vi "RT Main.vi"() -> ()   [LabVIEW 2014]
uses:
  <vilib>/addons/_NISVFA/_Shared subVIs/Controls/svc_Window.ctl
  <vilib>/addons/_NISVFA/_Shared subVIs/Controls/svc_Channel Info.ctl
  <vilib>/addons/_NISVFA/_Shared subVIs/Controls/svc_Engineering Units Text Ring.ctl
  <vilib>/addons/_NISVFA/_Shared subVIs/Controls/svc_Weighting Filter Text Ring.ctl
  <vilib>/NI/cRIO Wfm/ChannelConfig.ctl
  <vilib>/addons/Sound and Vibration/svt_Calibration/SVL Scale Voltage to EU (N Ch - 1 Info).vi
  <vilib>/addons/Sound and Vibration/svt_Calibration/SVL Scale Voltage to EU (1 Ch).vi
  <vilib>/addons/_NISVFA/_Shared subVIs/Common/svc_Set SV Channel Info.vi
  <vilib>/addons/_NISVFA/_Shared subVIs/Common/svc_Set SV Channel Info (variant).vi
  <vilib>/addons/_NISVFA/_Shared subVIs/Common/SVL Set dB Reference (variant).vi
  <vilib>/FPGAPlugInAG/sbRIO-9651/niLvFpga_Open_sbRIO-9651.vi
  <vilib>/rvi/interface/common/dynamic/niFpgaDynamicAddResources.vi
  <vilib>/FPGAPlugInAG/Dynamic/niLvFpga_Reset_Dynamic.vi
  <vilib>/FPGAPlugInAG/Dynamic/niLvFpga_Run_Dynamic.vi
  <vilib>/NI/cRIO Wfm/AcqRead(Wfm).vi
  <vilib>/addons/_NISVFA/_Shared subVIs/Common/svc_Engineering Units to Unit Label.vi
  <vilib>/addons/_NISVFA/_Shared subVIs/Common/svc_Compute Scale Factor to Convert V to EU.vi
  <vilib>/addons/_NISVFA/_Shared subVIs/Common/svc_Set dB ref if Pascal.vi
  <vilib>/addons/_NISVFA/_Shared subVIs/Common/svc_Caller VI Returned in Error Source.vi
  <vilib>/addons/_NISVFA/_Baseband FFT/SVFA Power Spectrum (N Ch).vi
  <vilib>/addons/_NISVFA/_Zoom FFT/SVFA Zoom Power Spectrum (N Ch).vi
  <vilib>/addons/_NISVFA/_Subset FFT/SVFA Power Spectrum Subset (N Ch).vi
  <vilib>/addons/_NISVFA/_Baseband FFT/SVFA FFT Spectrum (Mag-Phase) (N Ch).vi
  <vilib>/addons/_NISVFA/_Zoom FFT/SVFA Zoom FFT Spectrum (Mag-Phase) (N Ch).vi
  <vilib>/addons/_NISVFA/_Subset FFT/SVFA FFT Spectrum Subset (Mag-Phase) (N Ch).vi
  <vilib>/addons/_NISVFA/_Baseband FFT/SVFA Power Spectral Density (N Ch).vi
  <vilib>/addons/_NISVFA/_Zoom FFT/SVFA Zoom Power Spectral Density (N Ch).vi
  <vilib>/addons/_NISVFA/_Subset FFT/SVFA Power Spectral Density Subset (N Ch).vi
  <vilib>/FPGAPlugInAG/Dynamic/niLvFpga_Close_Dynamic.vi
  <vilib>/rvi/interface/nirviOpenFPGA/nirviOpenFPGA.xnode
  FPGA Bitfiles/SOMHands-ON_FPGATarget_FPGAMainSPIAPIwi_O70J1gyptM8.lvbitx
  FPGA Main_SPI API with Waveform Library.vi
  <vilib>/rvi/interface/nirviMethod/nirviMethod.xnode
  <vilib>/rvi/interface/nirviCloseFPGA/nirviCloseFPGA.xnode
  <vilib>/NI/cRIO Wfm/cRIO Wfm.lvlib
  <vilib>/addons/Sound and Vibration/svt_Calibration/SoundVib_Calibration.lvlib
panel:
  in  "channel info":T1={"sensor sensitivity [mV/EU]"=1000.0, "engineering units"=1, "dB reference [EU]"=1.0, "custom label"="EU", "weighting filter"=0, "pregain [dB]"=0.0} {"pregain [dB]" format="%.2f"; "weighting filter" items=["Linear", "A-weighting", "B-weighting", "C-weighting", "ITU-R 468-4", "Dolby", "CCITT", "C-message", "Wb", "Wc", "Wd", "We", "Wf", "Wh", "Wj", "Wk", "Wm", "AES17 20 kHz lowpass", "AES17 40 kHz lowpass", "AES17 20 kHz highpass", "AES17 40 kHz highpass"]; "dB reference [EU]" format="%^.1e"; "engineering units" items=["custom..."=0, "V"=1, "A"=21, "Pa"=2, "N"=20, "g"=3, "m/s^2"=4, "m/s"=5, "m"=6, "mm/s"=12, "mm"=13, "micron/s"=14, "micron"=15, "in/s^2"=7, "in/s"=8, "in"=9, "mil/s"=10, "mil"=11, "rad/s^2"=16, "rad/s"=17, "rad"=18, "deg/s^2"=26, "deg/s"=27, "deg"=28, "RPM"=22, "cycle/s^2"=23, "Hz"=24, "cycle"=25, "strain"=19]; "sensor sensitivity [mV/EU]" format="%.2f"}
  in  "scan rate [S/s]":u32=25000
  in  "quit":bool
  in  "window":T4=1 items=["None"=0, "Hanning"=1, "Hamming"=2, "Blackman-Harris"=3, "Exact Blackman"=4, "Blackman"=5, "Flat Top"=6, "4 Term B-Harris "=7, "7 Term B-Harris"=8, "Low Sidelobe"=9, "Force"=64, "Exponential"=65, "Blackman Nuttall"=11, "Triangle"=30, "Bartlett-Hanning"=31, "Bohman"=32, "Parzen"=33, "Welch"=34, "Kaiser"=60, "Dolph-Chebyshev"=61, "Gaussian"=62]
  in  "Graph Tab Control":T5(tab)
  out "Power spectrum":cluster{"f0":dbl, "df":dbl, "magnitude":dbl[]}[](graph)
  out "Phase":cluster{"f0":dbl, "df":dbl, "phase":dbl[]}[](graph)
  out "Magnitude":cluster{"f0":dbl, "df":dbl, "magnitude":dbl[]}[](graph)
  out "PSD":cluster{"f0":dbl, "df":dbl, "magnitude":dbl[]}[](graph)
  in  "dB On":bool=TRUE
  in  "FFT Type":enum32{"Baseband", "Zoom", "Subset"}(tab)
  out "frequency resolution [Hz]":dbl=50.0 format="%.2f"
  out "time record [ms]":dbl=20.0 format="%.2f"
  in  "zoom settings":T6={"frequency range"={"start frequency"=500.0, "stop frequency"=2000.0}, "window"=enum."Hanning", "number of lines"=400, "% overlap"=0.0} {"% overlap" min=0.0 max=99.0 step=10.0 format="%.2f"; "number of lines" min=1 step=1; "frequency range"."stop frequency" min=0.0 format="%.2f"; "frequency range"."start frequency" min=0.0 format="%.2f"}
  out "zoom FFT":dbl=2.500000055879356 format="%.2f"
  out "baseband FFT":dbl=50.0 format="%.2f"
  out "frequency resolution [Hz] Subset":dbl format="%.2f"
  out "time record [ms] Subset":dbl format="%.2f"
  in  "frequency range 2":T7={"start frequency"=200.0, "stop frequency"=2000.0} {"stop frequency" min=0.0 format="%.2f"; "start frequency" min=0.0 format="%.2f"}
  in  "number of samples":i32=2000 min=128
  out "averages completed":dbl
  out "done":bool
  in  "averaging mode":T8(ring)=enum."RMS averaging"
  in  "number of averages":u32=10
  in  "linear mode":enum16{"One shot", "Auto restart"}(ring)=enum."Auto restart"
  in  "weighting mode":enum16{"Linear", "Exponential"}(ring)=enum."Exponential"
  in  "restart 2":bool
  in  "Samples per Channel":i32=1000
  # "Channel Settings"
  # "Averaging Settings"
  # "Analysis Settings"
  # "VI Controls"
  # "Increase number of samples to improve frequency resolution (for a given sampling frequency)"
  # "frequency resolution [Hz]"
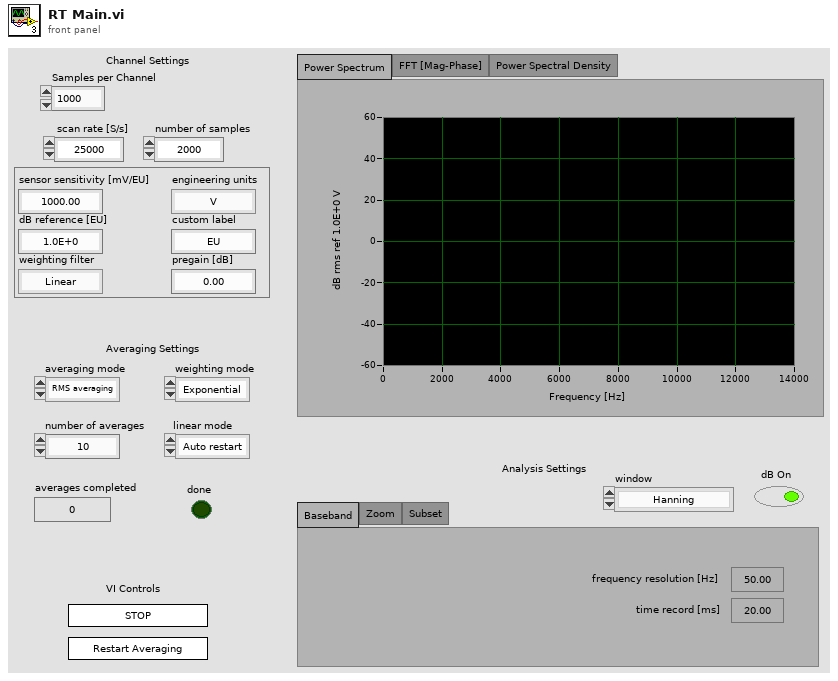
[diagram p1: front panel]
types:
  T1 = typedef "svc_Channel Info.ctl" = cluster{"sensor sensitivity [mV/EU]":dbl, "engineering units":T2, "dB reference [EU]":dbl, "custom label":string, "weighting filter":T3, "pregain [dB]":dbl}
  T2 = typedef "svc_Engineering Units Text Ring.ctl" = u16
  T3 = typedef "svc_Weighting Filter Text Ring.ctl" = u16
  T4 = typedef "svc_Window.ctl" = u32
  T5 = enum32{"Power Spectrum", "FFT [Mag-Phase]", "Power Spectral Density"}
  T6 = cluster{"frequency range":cluster{"start frequency":dbl, "stop frequency":dbl}, "window":enum16{"None ", "Hanning", "Hamming", "Blackman-Harris", "Exact Blackman", "Blackman", "Flat Top", "4 Term B-Harris ", "7 Term B-Harris", "Low Sidelobe"}, "number of lines":i32, "% overlap":dbl}
  T7 = cluster{"start frequency":dbl, "stop frequency":dbl}
  T8 = enum16{"No averaging", "Vector averaging", "RMS averaging", "Peak hold"}
  T9 = typedef "cRIO Wfm.lvlib/ChannelConfig.ctl" = cluster{"Channel Name":string, "Sensitivity mV_EU":dbl, "EU":string, "dB Ref EU":dbl}[]
  T10 = typedef "cRIO Wfm.lvlib/SamplingInfo.ctl" = cluster{"Number of Channels":i32, "Actual Samp Rate":dbl, "Chan Name Array":string[], "EU Chan Array":string[], "dB Ref Chan Array":dbl[]}
  T11 = cluster{"averaging mode":enum16{"No averaging", "Vector averaging", "RMS averaging", "Peak hold"}, "weighting mode":enum16{"Linear", "Exponential"}, "number of averages":u32, "linear mode":enum16{"One shot", "Auto restart"}}
  T12 = cluster{"dB On (T)":bool, "unwrap phase (F)":bool, "convert to degree (T)":bool}
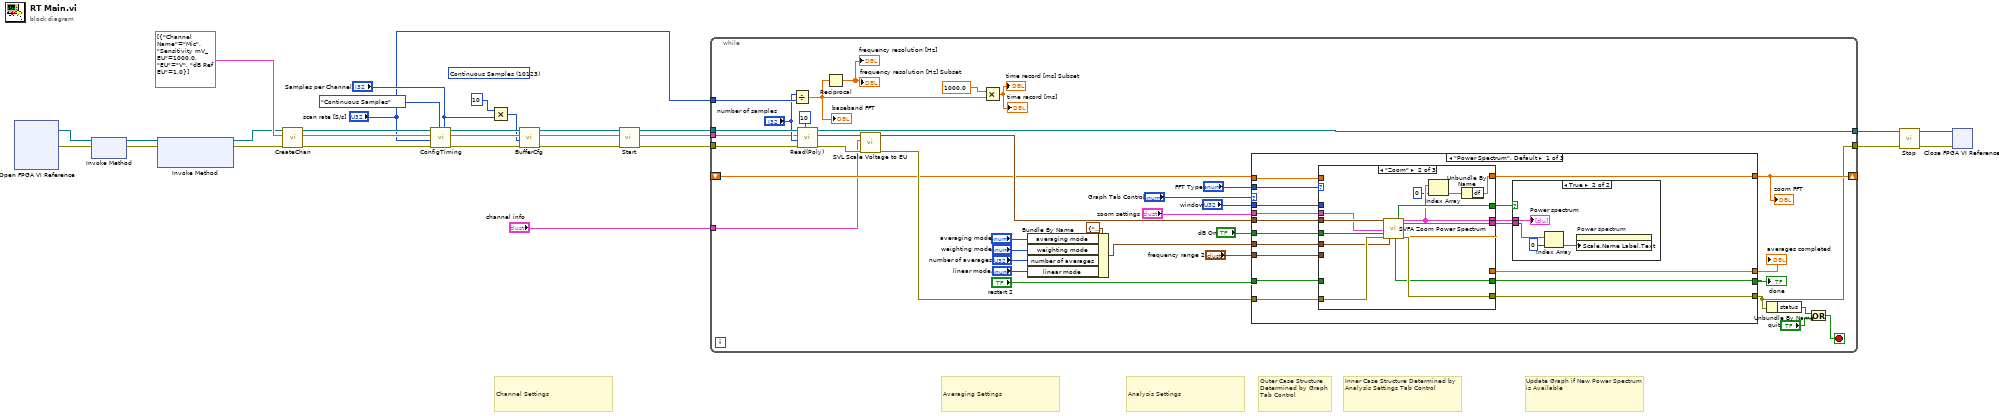
[diagram p0: block diagram]
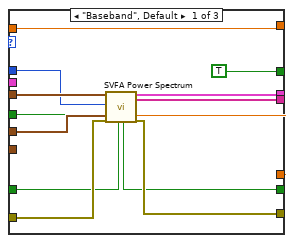
[diagram p3: hidden frame]
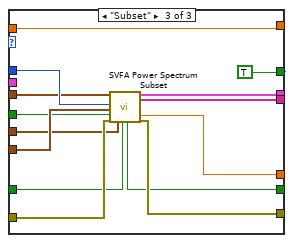
[diagram p4: hidden frame]
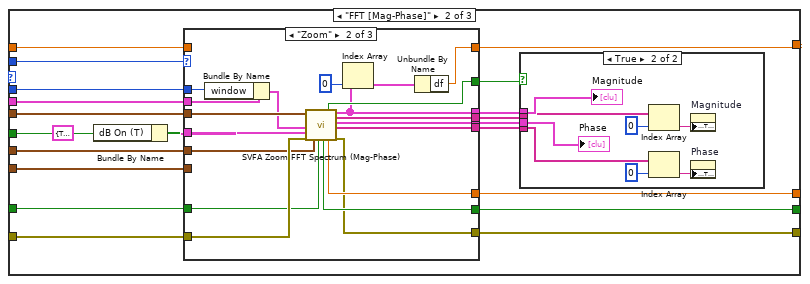
[diagram p5: hidden frame]
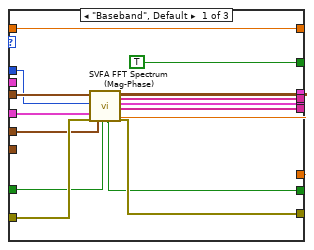
[diagram p7: hidden frame]
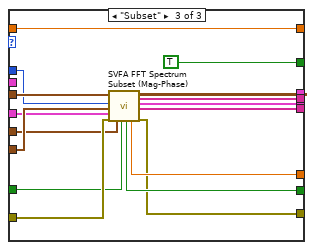
[diagram p8: hidden frame]
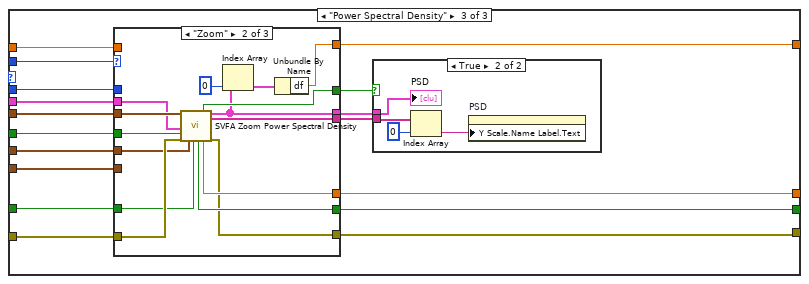
[diagram p9: hidden frame]
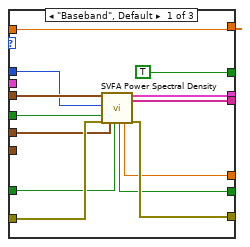
[diagram p11: hidden frame]
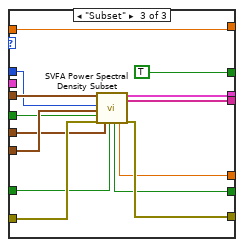
[diagram p12: hidden frame]
diagram:
  (unwired) 10123 items=["Finite Samples"=10178, "Continuous Samples"=10123] ("sample mode")
  # "Channel Settings"
  # "Update Graph if New Power Spectrum is Available"
  # "Inner Case Structure Determined by Analysis Settings Tab Control"
  # "Analysis Settings"
  # "Outer Case Structure Determined by Graph Tab Control"
  # "Averaging Settings"
  n1 = xnode "Open FPGA VI Reference"() -> ("FPGA VI Reference Out"=w15:refnum<k20>, "error out"=w16:errorcluster)  [unwired: 2 in]
  n2 = xnode "Invoke Method"("FPGA VI Reference In"=w15, "error in"=w16) -> ("FPGA VI Reference Out"=w14:refnum<k20>, "error out"=w11:errorcluster)
  n3 = xnode "Invoke Method"("FPGA VI Reference In"=w14, "error in"=w11) -> ("FPGA VI Reference Out"=w13:refnum<k20>, "error out"=w12:errorcluster)  [unwired: 1 in]
  n4 = call <vilib>:"CreateChan.vi"("error in"=w12, "Channel Info"=T9 [{"Channel Name"="Mic", "Sensitivity mV_EU"=1000.0, "EU"="V", "dB Ref EU"=1.0}], "Dynamic FPGA Ref"=w13) -> ("error out"=w19:errorcluster, "Sampling Info"=w23:T10, "Dynamic FPGA Ref Out"=w29:refnum<k20>)  [unwired: 6 in]
  n5 = call <vilib>:"ConfigTiming.vi"("Samples per Channel"="Samples per Channel", "Sample Mode"=enum16{"Finite Samples", "Continuous Samples"}."Continuous Samples", "error in"=w19, "Sample Rate"="scan rate [S/s]", "Sampling Info In"=w23, "Dynamic FPGA Ref"=w29) -> ("error out"=w18:errorcluster, "Sampling Info Out"=w24:T10, "Dynamic FPGA Ref Out"=w28:refnum<k20>)  [unwired: 2 in, 1 out]
  n6 = Multiply(x=10, y="Samples per Channel") -> (x*y=w20:i32)
  n7 = call <vilib>:"BufferCfg.vi"("error in"=w18, "Buffer Size [Samps per Chan]"=w20, "Sampling Info In"=w24, "Dynamic FPGA Ref"=w28) -> ("error out"=w17:errorcluster, "Sampling Info Out"=w22:T10, "Dynamic FPGA Ref Out"=w27:refnum<k20>)  [unwired: 4 in, 1 out]
  n8 = call <vilib>:"Start.vi"("error in"=w17, "Sampling Info In"=w22, "Dynamic FPGA Ref"=w27) -> ("error out"=w2:errorcluster, "Sampling Info Out"=w1:T10, "Dynamic FPGA Ref Out"=w3:refnum<k20>)  [unwired: 6 in]
  n9 = while {
    tunnel: [w32] -> w5
    shift-right: [w53] -> _
    shift-left: _ -> [w56]
    tunnel: [w48] -> w6
    tunnel: w3 -> [w47]
    tunnel: "scan rate [S/s]" -> [w46]
    tunnel: w2 -> [w43]
    tunnel: "channel info" -> [w34]
    tunnel: w1 -> [w30]
    stop <- w65 stop-if-true
    n10 = Divide(x="number of samples", y=w46) -> (x/y=w54:dbl)
    "baseband FFT" <- w54
    n11 = call-poly <vilib>:"Read(Poly).vi"("Poll Time (ms)"=u32 10, "error in"=w43, "Samps Read per Chan"="number of samples", "Sampling Info"=w30, "Dynamic FPGA Ref"=w47) -> ("error out"=w44:errorcluster, "Wfm Data"=w49:waveform(sgl)[], "Dynamic FPGA Ref Out"=w48:refnum<k20>)  [unwired: 3 in, 1 out]
    n12 = Reciprocal(x=w54) -> (1/x=→"frequency resolution [Hz]" →"frequency resolution [Hz] Subset":dbl)
    n13 = call-poly <vilib>:"SVL Scale Voltage to EU.vi"("error in (no error)"=w44, "channel info"=w34, "signals [V]"=w49) -> ("error out"=w64:errorcluster, "scaled signals [EU]"=w63:waveform(dbl)[])  [unwired: 6 in, 1 out]
    n14 = Multiply(x=1000.0 ("y"), y=w54) -> (x*y=→"time record [ms]" →"time record [ms] Subset":dbl)
    n15 = Bundle By Name(cluster=T11 {"averaging mode"=enum."RMS averaging", "weighting mode"=enum."Exponential", "number of averages"=10, "linear mode"=enum."Auto restart"} ("averaging parameters"), "averaging mode"="averaging mode", "weighting mode"="weighting mode", "number of averages"="number of averages", "linear mode"="linear mode") -> (w37:T11)
    n16 = case shown="\"Power Spectrum\", Default" "Graph Tab Control" {
      tunnel: w64 -> [w82 w149 w223]
      tunnel: w63 -> [w83 w148 w224]
      tunnel: [w81 w147 w222] -> w32
      tunnel: "window" -> [w80 w131 w221]
      tunnel: w37 -> [w79 w146 w220]
      tunnel: "restart 2" -> [w78 w145 w208]
      tunnel: [w76 w144 w219] -> w35
      tunnel: [w75 w143 w218] -> w36
      tunnel: "dB On" -> [w74 w141 w212]
      tunnel: "FFT Type" -> [w72 w136 w214]
      tunnel: [w71 w133 w211] -> w53
      tunnel: w56 -> [w69 w132 w210]
      tunnel: "zoom settings" -> [w68 w135 w213]
      tunnel: "frequency range 2" -> [w67 w130 w209]
      frame "Power Spectrum", Default {
        n17 = case shown="\"Zoom\"" w72 {
          tunnel: w83 -> [w100 w114 w126]
          tunnel: w82 -> [w99 w113 w125]
          tunnel: [w98 w112 w123] -> w81
          tunnel: w80 -> [w97 _ w127]
          tunnel: w79 -> [w96 w101 w115]
          tunnel: w78 -> [w95 _ w117]
          tunnel: [w94 w103 w124] -> w77
          tunnel: [w93 w107 w118] -> w76
          tunnel: [w92 w106 w119] -> w75
          tunnel: w74 -> [w91 w105 w116]
          tunnel: [w90 w109 w122] -> w73
          tunnel: [w88 w111 w120] -> w71
          tunnel: [TRUE ("new spectrum available") w110 TRUE ("new spectrum available")] -> w70
          tunnel: w69 -> [w88 _ w120]
          tunnel: w68 -> [_ w108 _]
          tunnel: w67 -> [_ _ w128]
          frame "Baseband", Default {
            n18 = call-poly <vilib>:"SVFA Power Spectrum.vi"("scaled signals [EU]"=w100, "window"=w97, "dB On (T)"=w91, "error in (no error)"=w99, "averaging parameters"=w96, "restart averaging (F)"=w95) -> ("averaging done"=w93:bool, "averages completed"=w92:dbl, "power spectra [dB EU]"=w94:cluster{"f0":dbl, "df":dbl, "magnitude":dbl[]}[], "unit labels"=w90:string[], "error out"=w98:errorcluster)  [unwired: 8 in, 1 out]
          }
          frame "Zoom" {
            n19 = call-poly <vilib>:"SVFA Zoom Power Spectrum.vi"("scaled signals [EU]"=w114, "zoom settings"=w108, "dB On (T)"=w105, "error in (no error)"=w113, "averaging parameters"=w101) -> ("averaging done"=w107:bool, "new spectrum available"=w110:bool, "averages completed"=w106:dbl, "power spectra [dB EU]"=w103:cluster{"f0":dbl, "df":dbl, "magnitude":dbl[]}[], "unit labels"=w109:string[], "error out"=w112:errorcluster)  [unwired: 8 in, 1 out]
            n20 = Index Array(array=w103, index=0) -> (element=w104:cluster{"f0":dbl, "df":dbl, "magnitude":dbl[]})
            n21 = Unbundle By Name(w104) -> ("df"=w111:dbl)
          }
          frame "Subset" {
            n22 = call-poly <vilib>:"SVFA Power Spectrum Subset.vi"("scaled signals [EU]"=w126, "window"=w127, "frequency range"=w128, "dB On (T)"=w116, "error in (no error)"=w125, "averaging parameters"=w115, "restart averaging (F)"=w117) -> ("averaging done"=w118:bool, "averages completed"=w119:dbl, "power spectra [dB EU]"=w124:cluster{"f0":dbl, "df":dbl, "magnitude":dbl[]}[], "unit labels"=w122:string[], "error out"=w123:errorcluster)  [unwired: 7 in, 1 out]
          }
        }
        n23 = case shown="True" w70 {
          tunnel: w77 -> [_ w87]
          tunnel: w73 -> [_ w86]
          frame False {
          }
          frame True {
            n24 = Index Array(array=w86, index=0) -> (element=w84:string)
            n25 = property on="Power spectrum" class="WFGraph (strict)"("Y Scale.Name Label.Text"=w84) -> ()  [unwired: 2 in, 2 out]
            "Power spectrum" <- w87
          }
        }
      }
      frame "FFT [Mag-Phase]" {
        n26 = Bundle By Name(cluster=T12 {"dB On (T)"=TRUE, "unwrap phase (F)"=FALSE, "convert to degree (T)"=TRUE} ("view"), "dB On (T)"=w141) -> (w140:T12)
        n27 = case shown="\"Zoom\"" w136 {
          tunnel: w149 -> [w172 w188 w206]
          tunnel: w148 -> [w171 w191 w207]
          tunnel: [w170 w184 w201] -> w147
          tunnel: w146 -> [w169 w187 w193]
          tunnel: w145 -> [w168 w178 w204]
          tunnel: [w167 w186 w203] -> w144
          tunnel: [w166 w185 w202] -> w143
          tunnel: w131 -> [w165 w176 w192]
          tunnel: [w164 w175 w200] -> w142
          tunnel: w140 -> [w163 w189 w196]
          tunnel: [w162 w182 w194] -> w129
          tunnel: [w161 w183 w197] -> w139
          tunnel: [w160 w181 w199] -> w137
          tunnel: w135 -> [_ w190 _]
          tunnel: [TRUE ("new spectrum available") w180 TRUE ("new spectrum available")] -> w134
          tunnel: [w158 w179 w195] -> w133
          tunnel: w132 -> [w158 _ w195]
          tunnel: w130 -> [_ _ w205]
          frame "Baseband", Default {
            n28 = call-poly <vilib>:"SVFA FFT Spectrum (Mag-Phase).vi"("scaled signals [EU]"=w171, "window"=w165, "view"=w163, "error in (no error)"=w172, "averaging parameters"=w169, "restart averaging (F)"=w168) -> ("averaging done"=w167:bool, "averages completed"=w166:dbl, "magnitudes [dB EU]"=w164:cluster{"f0":dbl, "df":dbl, "magnitude":dbl[]}[], "magnitude unit labels"=w161:string[], "phases [degrees]"=w162:cluster{"f0":dbl, "df":dbl, "phase":dbl[]}[], "phase unit labels"=w160:string[], "error out"=w170:errorcluster)  [unwired: 6 in, 1 out]
          }
          frame "Zoom" {
            n29 = Bundle By Name(cluster=w190, "window"=w176) -> (w177:T6)
            n30 = call-poly <vilib>:"SVFA Zoom FFT Spectrum (Mag-Phase).vi"("scaled signals [EU]"=w191, "zoom settings"=w177, "view"=w189, "error in (no error)"=w188, "averaging parameters"=w187, "restart averaging (F)"=w178) -> ("averaging done"=w186:bool, "new spectrum available"=w180:bool, "averages completed"=w185:dbl, "magnitudes [dB EU]"=w175:cluster{"f0":dbl, "df":dbl, "magnitude":dbl[]}[], "magnitude unit labels"=w183:string[], "phases [degrees]"=w182:cluster{"f0":dbl, "df":dbl, "phase":dbl[]}[], "phase unit labels"=w181:string[], "error out"=w184:errorcluster)  [unwired: 5 in, 1 out]
            n31 = Index Array(array=w175, index=0) -> (element=w174:cluster{"f0":dbl, "df":dbl, "magnitude":dbl[]})
            n32 = Unbundle By Name(w174) -> ("df"=w179:dbl)
          }
          frame "Subset" {
            n33 = call-poly <vilib>:"SVFA FFT Spectrum Subset (Mag-Phase).vi"("scaled signals [EU]"=w207, "window"=w192, "frequency range"=w205, "view"=w196, "error in (no error)"=w206, "averaging parameters"=w193, "restart averaging (F)"=w204) -> ("averaging done"=w203:bool, "averages completed"=w202:dbl, "magnitudes [dB EU]"=w200:cluster{"f0":dbl, "df":dbl, "magnitude":dbl[]}[], "magnitude unit labels"=w197:string[], "phases [degrees]"=w194:cluster{"f0":dbl, "df":dbl, "phase":dbl[]}[], "phase unit labels"=w199:string[], "error out"=w201:errorcluster)  [unwired: 5 in, 1 out]
          }
        }
        n34 = case shown="True" w134 {
          tunnel: w142 -> [_ w157]
          tunnel: w139 -> [_ w152]
          tunnel: w137 -> [_ w155]
          tunnel: w129 -> [_ w156]
          frame False {
          }
          frame True {
            n35 = Index Array(array=w152, index=0) -> (element=w150:string)
            n36 = Index Array(array=w155, index=0) -> (element=w153:string)
            n37 = property on="Magnitude" class="WFGraph (strict)"("Y Scale.Name Label.Text"=w150) -> ()  [unwired: 2 in, 2 out]
            n38 = property on="Phase" class="WFGraph (strict)"("Y Scale.Name Label.Text"=w153) -> ()  [unwired: 2 in, 2 out]
            "Magnitude" <- w157
            "Phase" <- w156
          }
        }
      }
      frame "Power Spectral Density" {
        n39 = case shown="\"Zoom\"" w214 {
          tunnel: w224 -> [w241 w256 w269]
          tunnel: w223 -> [w240 w255 w262]
          tunnel: [w239 w248 w270] -> w222
          tunnel: w221 -> [w238 _ w261]
          tunnel: w220 -> [w237 w252 w258]
          tunnel: w208 -> [w236 w251 w257]
          tunnel: [w235 w250 w263] -> w219
          tunnel: [w234 w249 w264] -> w218
          tunnel: [w233 w244 w267] -> w217
          tunnel: [w232 w247 w266] -> w216
          tunnel: [TRUE ("new spectrum available") w246 TRUE ("new spectrum available")] -> w215
          tunnel: w213 -> [_ w254 _]
          tunnel: w212 -> [w229 w253 w259]
          tunnel: [w231 w245 w268] -> w211
          tunnel: w210 -> [w231 _ w268]
          tunnel: w209 -> [_ _ w260]
          frame "Baseband", Default {
            n40 = call-poly <vilib>:"SVFA Power Spectral Density.vi"("scaled signals [EU]"=w241, "window"=w238, "dB On (F)"=w229, "error in (no error)"=w240, "averaging parameters"=w237, "restart averaging (F)"=w236) -> ("averaging done"=w235:bool, "averages completed"=w234:dbl, "power spectral densities [EU^2 rms / Hz]"=w233:cluster{"f0":dbl, "df":dbl, "magnitude":dbl[]}[], "unit labels"=w232:string[], "error out"=w239:errorcluster)  [unwired: 8 in, 1 out]
          }
          frame "Zoom" {
            n41 = call-poly <vilib>:"SVFA Zoom Power Spectral Density.vi"("scaled signals [EU]"=w256, "zoom settings"=w254, "dB On (T)"=w253, "error in (no error)"=w255, "averaging parameters"=w252, "restart averaging (F)"=w251) -> ("averaging done"=w250:bool, "new spectrum available"=w246:bool, "averages completed"=w249:dbl, "power spectral densities [EU^2 rms / Hz]"=w244:cluster{"f0":dbl, "df":dbl, "magnitude":dbl[]}[], "unit labels"=w247:string[], "error out"=w248:errorcluster)  [unwired: 7 in, 1 out]
            n42 = Index Array(array=w244, index=0) -> (element=w243:cluster{"f0":dbl, "df":dbl, "magnitude":dbl[]})
            n43 = Unbundle By Name(w243) -> ("df"=w245:dbl)
          }
          frame "Subset" {
            n44 = call-poly <vilib>:"SVFA Power Spectral Density Subset.vi"("scaled signals [EU]"=w269, "window"=w261, "frequency range"=w260, "dB On (T)"=w259, "error in (no error)"=w262, "averaging parameters"=w258, "restart averaging (F)"=w257) -> ("averaging done"=w263:bool, "averages completed"=w264:dbl, "power spectral densities [EU^2 rms / Hz]"=w267:cluster{"f0":dbl, "df":dbl, "magnitude":dbl[]}[], "unit labels"=w266:string[], "error out"=w270:errorcluster)  [unwired: 7 in, 1 out]
          }
        }
        n45 = case shown="True" w215 {
          tunnel: w217 -> [_ w228]
          tunnel: w216 -> [_ w227]
          frame False {
          }
          frame True {
            n46 = Index Array(array=w227, index=0) -> (element=w225:string)
            n47 = property on="PSD" class="WFGraph (strict)"("Y Scale.Name Label.Text"=w225) -> ()  [unwired: 2 in, 2 out]
            "PSD" <- w228
          }
        }
      }
    }
    "zoom FFT" <- w53
    "averages completed" <- w36
    "done" <- w35
    n48 = Unbundle By Name(w32) -> ("status"=w62:bool)
    n49 = Or(x=w62, y="quit") -> (x .or. y?=w65:bool)
  }
  n50 = call <vilib>:"Stop.vi"("error in"=w5, "Dynamic FPGA Ref"=w6) -> ("error out"=w9:errorcluster, "Dynamic FPGA Ref Out"=w10:refnum<k20>)  [unwired: 8 in]
  n51 = xnode "Close FPGA VI Reference"("FPGA VI Reference In"=w10, "error in"=w9) -> ()  [unwired: 1 out]
